vi "GetMethodName.vi"(8 "error in (no error)":errorcluster, 11 "VI Reference":refnum<vi>) -> (0 "error out":errorcluster, 2 "Method Name":string, 3 "VI Reference out":refnum<vi>)   [LabVIEW 2017, in "DynamicDispatchImplementationWalker.lvlib"]
uses:
  DynamicDispatchImplementationWalker.lvlib
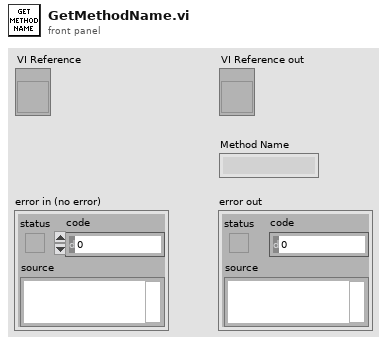
[diagram p1: front panel]
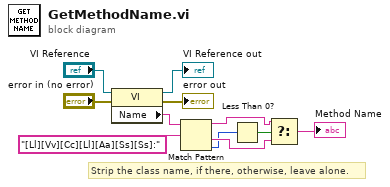
[diagram p0: block diagram]
diagram:
  # "Strip the class name, if there, otherwise, leave alone."
  n1 = property class="VI"(reference="VI Reference", error in="error in (no error)") -> (reference out=→"VI Reference out":refnum<vi>, error out=→"error out":errorcluster, "Name"=w1:string)
  n2 = Match Pattern(string=w1, regular expression="[Ll][Vv][Cc][Ll][Aa][Ss][Ss]:") -> (before substring=w6:string, after substring=w7:string, offset past match=w4:i32)  [unwired: 1 in, 1 out]
  n3 = Less Than 0?(x=w4) -> (x < 0?=w5:bool)
  n4 = Select(t=w6, s=w5, f=w7) -> (s? t:f=→"Method Name":string)
